vi "FFValid.vi"(7 "error in (no error)":errorcluster, 10 "drv":u32=1) -> (0 "error out":errorcluster, 3 "FFvalid":u8)   [LabVIEW 2015, in "ESLSCDLL.lvlib"]
uses:
  ESLSCDLL.lvlib
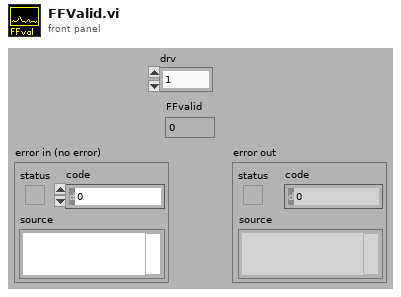
[diagram p1: front panel]
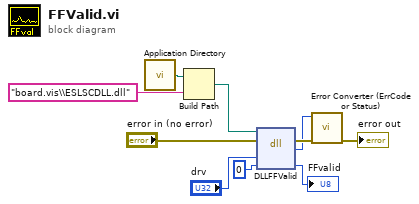
[diagram p0: block diagram]
diagram:
  n1 = call <vilib>:"Application Directory.vi"() -> ("Application Directory"=w3:path)
  n2 = Build Path(base path=w3, name or relative path="board.vis\\ESLSCDLL.dll") -> (appended path=w1:path)
  n3 = dll-call lib="C:/ENTW/PCIE/LV64/board.vis/ESLSCDLL.dll" fn="DLLFFValid"(path in=w1, error in="error in (no error)", "drv"="drv", "valid"=u8 0) -> (error out=w6:errorcluster, "es_status_codes"=w5:i32, "valid"=→"FFvalid":u8)  [unwired: 2 in, 1 out]
  n4 = call "Error Converter (ErrCode or Status).vi"("error in (no error)"=w6, "error code"=w5) -> ("error out"=→"error out":errorcluster)  [unwired: 9 in]
